vi "KM_messaround V2.vi.vi"() -> ()   [LabVIEW 2016]
uses:
  KM_SystemParameters.ctl
  KM_ControlHFLIcommand.ctl
panel:
  in  "Control HFLI command":T1=enum."Scan frequency"
  in  "ZI HFLI System Parameters IN":T2={"IP Address"="DEV3523", "Start (Hz)"=44300.0, "Stop (Hz)"=44600.0, "Filter Order"=4, "Number of Points"=100, "Precision"=0, "Bandwidth (Hz)"=50.0, "Averaging"=1, "Log Sweep"=FALSE, "Demod"=0} {"Averaging" items=["1"=1, "2"=2, "4"=4, "16"=16, "32"=32, "64"=64]; "Bandwidth (Hz)" format="%#_p"; "Precision" items=["Low", "Med", "High"]; "Number of Points" min=2 max=66000; "Filter Order" items=["6, 1st"=1, "12, 2nd"=2, "18, 3rd"=3, "24, 4th"=4, "30, 5th"=5, "36, 6th"=6, "42, 7th"=7, "48, 8th"=8]; "Stop (Hz)" format="%_5p"; "Start (Hz)" format="%_5p"}
  out "Plot: All 2":cluster{dbl[], dbl[]}(graph)={[-2.0402873565910927e-06, -1.9543192329064616e-06, 6.181317276778432e-07, 2.0293344232366778e-06, 2.0560936177205287e-06, 1.646227433562011e-06, 1.2185597511767214e-06, 8.799812537335215e-07, 2.658072034660254e-07, -1.1163727231853217e-07, -4.237225273835034e-07, -6.57452090558403e-07, -1.4840300422219474e-06, -1.860129849849155e-06, -2.768328264206093e-06, -2.8791569467147063e-06, -3.7399425407350324e-06, -4.205436841551143e-06, -4.7947002433604135e-06, -5.216462715651585e-06, -6.102833975582075e-06, -6.49309603098625e-06, -7.497123667616776e-06, -7.82070509004563e-06, -8.929863713289655e-06, -9.346845010731321e-06, -9.766975992078586e-06, -1.0548320618800247e-05, -1.1614953142572177e-05, -1.1969749948016977e-05, -1.3065918063142214e-05, -1.3468102047801335e-05, -1.4545386967122222e-05, -1.5220863574040812e-05, -1.5836207575050978e-05, -1.6306476491359728e-05, -1.749714764606146e-05, -1.9441456704086576e-05, -1.903958399072596e-05, -2.176326032753049e-05, -2.053816268647475e-05, -2.3289644137030532e-05, -2.5551851829218626e-05, -2.5848313888841213e-05, -2.6824957403170194e-05, -2.8036811702715253e-05, -3.0228989315790625e-05, -3.17046627373664e-05, -3.149898575458813e-05, -3.383422234458664e-05, -3.624554985944125e-05, -3.7025401338018346e-05, -3.92908475635823e-05, -4.269987651352361e-05, -4.400525531586193e-05, -4.724242255658017e-05, -4.986033164915528e-05, -5.269880925350801e-05, -5.555267451276114e-05, -6.098681604533867e-05, -6.504986475328242e-05, -6.891726036834814e-05, -7.392144559929962e-05, -8.14138858861147e-05, -8.858387832662824e-05, -9.434564184546356e-05, -0.00010299581160049854, -0.0001181276557573021, -0.00013007532213966973, -0.00014515893653805438, -0.00016084591457028765, -0.00019370365619185661, -0.00022071482717707074, -0.0002549125261451503, -0.00030280456951649706, -0.0003902313528436058, -0.0004818229568782516, -0.0006001535752372003, -0.0007678749957474056, -0.001004875218835482, -0.0011526629494206765, -0.0011474676966836009, -0.0009344314709005343, -0.0005784531702449823, -0.0003819260800355906, -0.00025311777280887063, -0.0001712735012814078, -0.00010500601178345449, -7.433080730928469e-05, -5.529514521765891e-05, -3.723578555380511e-05, -2.4617963991852023e-05, -1.7465616817610815e-05, -1.1968715954852966e-05, -8.078403139510855e-06, -3.2853123238030737e-06, -3.057427147594998e-06, -5.63415957929672e-07, 9.25684467149015e-07, 1.334252494953408e-06], [0.0007363464237155247, 0.0007366592322887604, 0.0007857482074227841, 0.0008143543945572935, 0.0008237259570136081, 0.0008296961894160256, 0.0008358289209401988, 0.0008413996777760374, 0.0008487849202825212, 0.0008537411739076386, 0.0008590566137405538, 0.0008634596547854978, 0.0008697415448921736, 0.0008739729394940608, 0.0008783010380979052, 0.0008821410698650452, 0.0008871648437208166, 0.0008909225955117455, 0.0008946744647521769, 0.0008979893162451642, 0.0009028400781190406, 0.00090600256946707, 0.000909415810120424, 0.0009126006587381756, 0.0009171621440297225, 0.0009203489908660974, 0.0009237561026949185, 0.0009266651494382574, 0.0009308699052993048, 0.0009337095397356865, 0.0009371409533853877, 0.0009403100655097149, 0.0009437772866885428, 0.0009469982129616631, 0.000949974626088922, 0.0009534209014523642, 0.0009581719986691163, 0.0009614544165276263, 0.0009634966991213149, 0.0009684521990166979, 0.0009714214212999172, 0.0009743132163383956, 0.0009790413331465231, 0.0009833951026879172, 0.0009887311639462059, 0.000992377202137755, 0.0009956339275917292, 0.0009981972580647453, 0.0010034254262508752, 0.0010093361772126296, 0.0010121011268117448, 0.001018100284785327, 0.0010230503702297704, 0.0010289127858870907, 0.001034406406475111, 0.0010418517511759395, 0.0010478383670628904, 0.0010540190194594048, 0.0010601439769530828, 0.001069647350281907, 0.0010765128603582677, 0.0010850662927182556, 0.001093822865975136, 0.0011070706225292932, 0.0011172477992327304, 0.0011265500841470563, 0.0011395582625769356, 0.0011588366161021295, 0.0011733869267610366, 0.001190598026817262, 0.00120894005182803, 0.0012371184788528531, 0.001259456436039511, 0.001285500271834093, 0.0013158647237952517, 0.0013472354639859387, 0.0013716173155791584, 0.0013838373354031434, 0.0013508967723602698, 0.0011845081791756623, 0.0009245586411999766, 0.0005830080931981382, 0.00028800273316293464, 0.00017750561183252903, 0.00022692326023882444, 0.00029992873577849226, 0.0003728646314494504, 0.00045244150862236036, 0.0005079265549732318, 0.0005474404355778574, 0.0005844424140488156, 0.0006246993302508499, 0.0006497210900402344, 0.0006718457685458125, 0.0006906838377638436, 0.0007148351058999629, 0.0007293483526147512, 0.0007422883256593365, 0.0007560103845379693, 0.000769240281155993]}
  in  "df 2":dbl=100.0
  in  "freq max 2":dbl=50000.0
  in  "freq min 2":dbl=40000.0
  out "Plot: All":cluster{dbl[], dbl[]}[](graph)=[{[41267.16294185641, 43382.62629568044, 43809.54524796477, 43993.158550466134, 44095.48866448749, 44160.83178737423, 44206.24620896132, 44239.69869830655, 44265.409282963716, 44285.82217210024, 44302.45097954066, 44316.283154692006, 44327.99036525239, 44338.045411679006, 44346.790780314026, 44354.480668671866, 44361.30773369069, 44367.420672012246, 44372.93610031889, 44377.946781345774, 44382.52744309405, 44386.73897468617, 44390.63150381164, 44394.24668885297, 44397.61945004213, 44400.779293629195, 44403.75133657101, 44406.55710798093, 44409.21518218587, 44411.74168336905, 44414.15069129511, 44416.45457012791, 44418.664236937904, 44420.789382536845, 44422.83865435258, 44424.81980887248, 44426.73983954013, 44428.605084740426, 44430.42131955211, 44432.19383420931, 44433.92750164089, 44435.62683600951, 44437.296043821305, 44438.93906889986, 44440.55963229991, 44442.16126806206, 44443.747355572785, 44445.321149185525, 44446.88580567351, 44448.44441001973, 44450.0, 44451.55558998027, 44453.11419432649, 44454.678850814475, 44456.252644427215, 44457.83873193794, 44459.44036770009, 44461.06093110014, 44462.703956178695, 44464.37316399049, 44466.07249835911, 44467.80616579069, 44469.57868044789, 44471.394915259574, 44473.26016045987, 44475.18019112752, 44477.16134564742, 44479.210617463155, 44481.335763062096, 44483.54542987209, 44485.84930870489, 44488.25831663095, 44490.78481781413, 44493.44289201907, 44496.24866342899, 44499.220706370805, 44502.38054995787, 44505.75331114703, 44509.36849618836, 44513.26102531383, 44517.47255690595, 44522.053218654226, 44527.06389968111, 44532.579327987754, 44538.69226630931, 44545.519331328134, 44553.209219685974, 44561.954588320994, 44572.00963474761, 44583.716845307994, 44597.54902045934, 44614.17782789976, 44634.590717036284, 44660.30130169345, 44693.75379103868, 44739.16821262577, 44804.51133551251, 44906.841449533866, 45090.45475203523, 45517.37370431956], [-2.0402873565910927e-06, -1.9543192329064616e-06, 6.181317276778432e-07, 2.0293344232366778e-06, 2.0560936177205287e-06, 1.646227433562011e-06, 1.2185597511767214e-06, 8.799812537335215e-07, 2.658072034660254e-07, -1.1163727231853217e-07, -4.237225273835034e-07, -6.57452090558403e-07, -1.4840300422219474e-06, -1.860129849849155e-06, -2.768328264206093e-06, -2.8791569467147063e-06, -3.7399425407350324e-06, -4.205436841551143e-06, -4.7947002433604135e-06, -5.216462715651585e-06, -6.102833975582075e-06, -6.49309603098625e-06, -7.497123667616776e-06, -7.82070509004563e-06, -8.929863713289655e-06, -9.346845010731321e-06, -9.766975992078586e-06, -1.0548320618800247e-05, -1.1614953142572177e-05, -1.1969749948016977e-05, -1.3065918063142214e-05, -1.3468102047801335e-05, -1.4545386967122222e-05, -1.5220863574040812e-05, -1.5836207575050978e-05, -1.6306476491359728e-05, -1.749714764606146e-05, -1.9441456704086576e-05, -1.903958399072596e-05, -2.176326032753049e-05, -2.053816268647475e-05, -2.3289644137030532e-05, -2.5551851829218626e-05, -2.5848313888841213e-05, -2.6824957403170194e-05, -2.8036811702715253e-05, -3.0228989315790625e-05, -3.17046627373664e-05, -3.149898575458813e-05, -3.383422234458664e-05, -3.624554985944125e-05, -3.7025401338018346e-05, -3.92908475635823e-05, -4.269987651352361e-05, -4.400525531586193e-05, -4.724242255658017e-05, -4.986033164915528e-05, -5.269880925350801e-05, -5.555267451276114e-05, -6.098681604533867e-05, -6.504986475328242e-05, -6.891726036834814e-05, -7.392144559929962e-05, -8.14138858861147e-05, -8.858387832662824e-05, -9.434564184546356e-05, -0.00010299581160049854, -0.0001181276557573021, -0.00013007532213966973, -0.00014515893653805438, -0.00016084591457028765, -0.00019370365619185661, -0.00022071482717707074, -0.0002549125261451503, -0.00030280456951649706, -0.0003902313528436058, -0.0004818229568782516, -0.0006001535752372003, -0.0007678749957474056, -0.001004875218835482, -0.0011526629494206765, -0.0011474676966836009, -0.0009344314709005343, -0.0005784531702449823, -0.0003819260800355906, -0.00025311777280887063, -0.0001712735012814078, -0.00010500601178345449, -7.433080730928469e-05, -5.529514521765891e-05, -3.723578555380511e-05, -2.4617963991852023e-05, -1.7465616817610815e-05, -1.1968715954852966e-05, -8.078403139510855e-06, -3.2853123238030737e-06, -3.057427147594998e-06, -5.63415957929672e-07, 9.25684467149015e-07, 1.334252494953408e-06]}, {[41267.16294185641, 43382.62629568044, 43809.54524796477, 43993.158550466134, 44095.48866448749, 44160.83178737423, 44206.24620896132, 44239.69869830655, 44265.409282963716, 44285.82217210024, 44302.45097954066, 44316.283154692006, 44327.99036525239, 44338.045411679006, 44346.790780314026, 44354.480668671866, 44361.30773369069, 44367.420672012246, 44372.93610031889, 44377.946781345774, 44382.52744309405, 44386.73897468617, 44390.63150381164, 44394.24668885297, 44397.61945004213, 44400.779293629195, 44403.75133657101, 44406.55710798093, 44409.21518218587, 44411.74168336905, 44414.15069129511, 44416.45457012791, 44418.664236937904, 44420.789382536845, 44422.83865435258, 44424.81980887248, 44426.73983954013, 44428.605084740426, 44430.42131955211, 44432.19383420931, 44433.92750164089, 44435.62683600951, 44437.296043821305, 44438.93906889986, 44440.55963229991, 44442.16126806206, 44443.747355572785, 44445.321149185525, 44446.88580567351, 44448.44441001973, 44450.0, 44451.55558998027, 44453.11419432649, 44454.678850814475, 44456.252644427215, 44457.83873193794, 44459.44036770009, 44461.06093110014, 44462.703956178695, 44464.37316399049, 44466.07249835911, 44467.80616579069, 44469.57868044789, 44471.394915259574, 44473.26016045987, 44475.18019112752, 44477.16134564742, 44479.210617463155, 44481.335763062096, 44483.54542987209, 44485.84930870489, 44488.25831663095, 44490.78481781413, 44493.44289201907, 44496.24866342899, 44499.220706370805, 44502.38054995787, 44505.75331114703, 44509.36849618836, 44513.26102531383, 44517.47255690595, 44522.053218654226, 44527.06389968111, 44532.579327987754, 44538.69226630931, 44545.519331328134, 44553.209219685974, 44561.954588320994, 44572.00963474761, 44583.716845307994, 44597.54902045934, 44614.17782789976, 44634.590717036284, 44660.30130169345, 44693.75379103868, 44739.16821262577, 44804.51133551251, 44906.841449533866, 45090.45475203523, 45517.37370431956], [0.0007363464237155247, 0.0007366592322887604, 0.0007857482074227841, 0.0008143543945572935, 0.0008237259570136081, 0.0008296961894160256, 0.0008358289209401988, 0.0008413996777760374, 0.0008487849202825212, 0.0008537411739076386, 0.0008590566137405538, 0.0008634596547854978, 0.0008697415448921736, 0.0008739729394940608, 0.0008783010380979052, 0.0008821410698650452, 0.0008871648437208166, 0.0008909225955117455, 0.0008946744647521769, 0.0008979893162451642, 0.0009028400781190406, 0.00090600256946707, 0.000909415810120424, 0.0009126006587381756, 0.0009171621440297225, 0.0009203489908660974, 0.0009237561026949185, 0.0009266651494382574, 0.0009308699052993048, 0.0009337095397356865, 0.0009371409533853877, 0.0009403100655097149, 0.0009437772866885428, 0.0009469982129616631, 0.000949974626088922, 0.0009534209014523642, 0.0009581719986691163, 0.0009614544165276263, 0.0009634966991213149, 0.0009684521990166979, 0.0009714214212999172, 0.0009743132163383956, 0.0009790413331465231, 0.0009833951026879172, 0.0009887311639462059, 0.000992377202137755, 0.0009956339275917292, 0.0009981972580647453, 0.0010034254262508752, 0.0010093361772126296, 0.0010121011268117448, 0.001018100284785327, 0.0010230503702297704, 0.0010289127858870907, 0.001034406406475111, 0.0010418517511759395, 0.0010478383670628904, 0.0010540190194594048, 0.0010601439769530828, 0.001069647350281907, 0.0010765128603582677, 0.0010850662927182556, 0.001093822865975136, 0.0011070706225292932, 0.0011172477992327304, 0.0011265500841470563, 0.0011395582625769356, 0.0011588366161021295, 0.0011733869267610366, 0.001190598026817262, 0.00120894005182803, 0.0012371184788528531, 0.001259456436039511, 0.001285500271834093, 0.0013158647237952517, 0.0013472354639859387, 0.0013716173155791584, 0.0013838373354031434, 0.0013508967723602698, 0.0011845081791756623, 0.0009245586411999766, 0.0005830080931981382, 0.00028800273316293464, 0.00017750561183252903, 0.00022692326023882444, 0.00029992873577849226, 0.0003728646314494504, 0.00045244150862236036, 0.0005079265549732318, 0.0005474404355778574, 0.0005844424140488156, 0.0006246993302508499, 0.0006497210900402344, 0.0006718457685458125, 0.0006906838377638436, 0.0007148351058999629, 0.0007293483526147512, 0.0007422883256593365, 0.0007560103845379693, 0.000769240281155993]}]
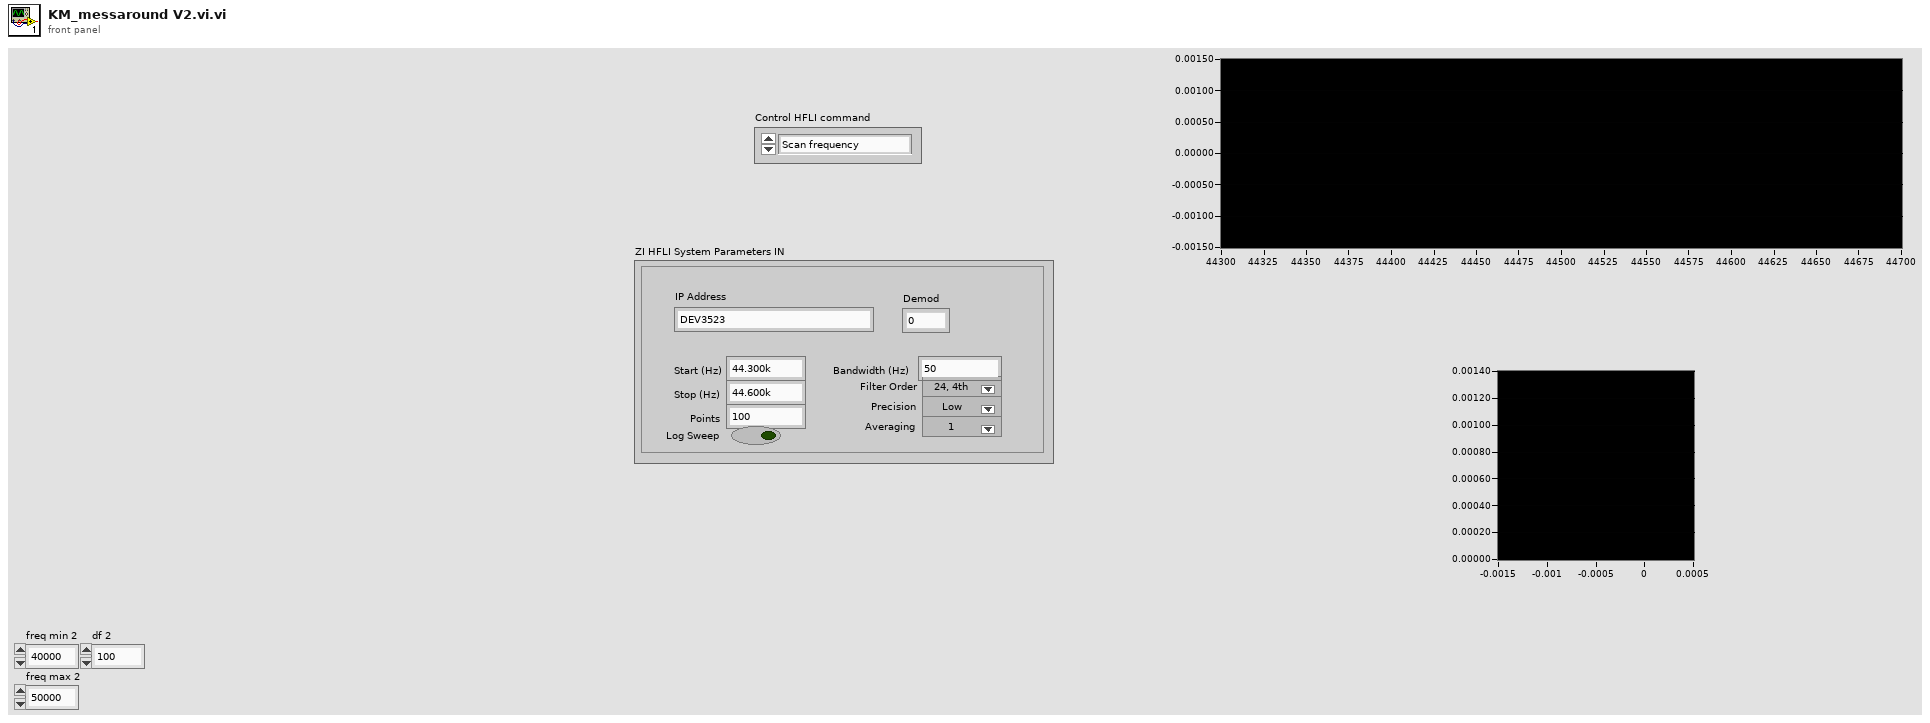
[diagram p1: front panel]
types:
  T1 = typedef "KM_ControlHFLIcommand.ctl" = enum16{"Initialize", "Scan frequency"}
  T2 = typedef "KM_SystemParameters.ctl" = cluster{"IP Address":string, "Start (Hz)":dbl, "Stop (Hz)":dbl, "Filter Order":i32, "Number of Points":i32, "Precision":u16, "Bandwidth (Hz)":dbl, "Averaging":u16, "Log Sweep":bool, "Demod":i32}
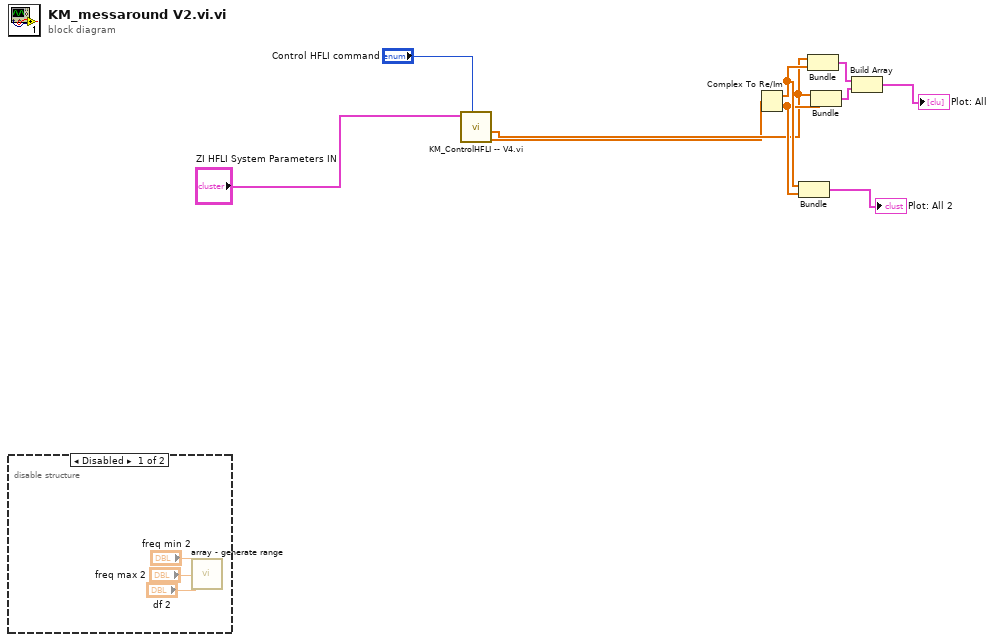
[diagram p0: block diagram]
diagram:
  n1 = disable-structure shown="Disabled" {
    frame Disabled {
      n2 = call "array - generate range.vi"("df"="df 2", "freq max"="freq max 2", "freq min"="freq min 2") -> ()  [unwired: 7 in, 2 out]
    }
    frame Enabled {
    }
  }
  n3 = call "KM_ControlHFLI -- V4.vi.vi"("Control HFLI command"="Control HFLI command", "ZI HFLI System Parameters IN"="ZI HFLI System Parameters IN") -> ("Voltage out"=w1:cdb[], "Freq out"=w2:dbl[])  [unwired: 4 in, 1 out]
  n4 = Complex To Re/Im(x + iy=w1) -> (x=w7:dbl[], y=w6:dbl[])
  n5 = Bundle(w7, w6) -> (→"Plot: All 2":cluster{dbl[], dbl[]})  [unwired: 1 in]
  n6 = Bundle("Freq out"=w2, w7) -> (w10:cluster{"Freq out":dbl[], dbl[]})  [unwired: 1 in]
  n7 = Bundle("Freq out"=w2, w6) -> (w9:cluster{"Freq out":dbl[], dbl[]})  [unwired: 1 in]
  n8 = Build Array(w10, w9) -> (→"Plot: All":cluster{"Freq out":dbl[], dbl[]}[])
